vi "2100_Test_Set State_Measure Resistance_Source and Sink.vi"(0 "Semiconductor Module Context":T7, 1 "Script_Info":T3={"Script Name"="WalkingState", "All_Scripts"=[]}, 2 "current range":dbl=1e-05 format="%#_6p", 3 "current level":dbl=1e-05 format="%#_13p", 4 "Instrument_Pins":T6={"SMU_Pins"=["RF1", "RF2", "RF3", "RF4"], "HSDIO_Pins"=["CLK", "SDA"]}, 5 "Error In":errorcluster, 6 "USID":T4, 7 "Master_Register_Data_Array_In":T1 {"Address" format="%.0x"}, 10 "Publishable IDs":string[](array[string])=["RF1", "RF2", "RF3", "RF4"], 11 "Reg_Map_and_Bit_Name":T5={"Reg_Map_Bit_Name"="", "Reg_Map"=[["Reg Addr(0x00)", "7", "6", "5", "4", "3", "2", "1", "0"], ["0", "SPARE", "RF3_SH", "RF2_SH", "RF1_SH", "SPARE", "RF3_RFC", "RF2_RFC", "RF1_RFC"], ["1", "SPARE[7:0]", "", "", "", "", "", "", ""], ["2", "VVAR_EN", "LCM_EN", "RFC_SH", "SPARE", "VARACTOR[3:0]", "", "", ""], ["3", "SW_CTRL1_VIRTUAL[7:0]", "", "", "", "", "", "", ""], ["4", "SW_CTRL1_SWAP", "SW_CTRL1_RBSHIFT[2:0]", "", "", "SW_CTRL1_VSID[3:0]", "", "", ""], ["5", "REG_00_VIRTUAL_MASK[7:0]", "", "", "", "", "", "", ""], ["6", "LOCK_STATUS[1:0]", "", "CLK_DITHER", "FUSES_BURNED", "CLK_IDAC_CAL[3:0]", "", "", ""], ["7", "SPARE[2:0]", "", "", "ODFT_TRIM[4:0]", "", "", "", ""], ["8", "SPARE[2:0]", "", "", "HV_TRIM[4:0]", "", "", "", ""], ["9", "TEST_MUX[2:0]", "", "", "SPARE[1:0]", "", "MEMS_BG_TC[1:0]", "", "MEMSCP_RCM"], ["A", "CP_BOOST_OVRD_EN", "SPARE[2:0]", "", "", "PS_OFF_TIMER[1:0]", "", "PS_ON_TIMER[1:0]", ""], ["0", "", "", "", "", "", "", "", ""], ["D", "Reserved[1:0]", "", "WD_HI_EVENT_CNT[5:0]", "", "", "", "", ""], ["E", "VERSION_ID[7:0]", "", "", "", "", "", "", ""], ["F", "Reserved", "COUNT_200_LSB[6:0]", "", "", "", "", "", ""], ["10", "CLK_DIV2_EN", "Spare", "ODFT_EN", "HV_HYST[4:0]", "", "", "", ""], ["0", "", "", "", "", "", "", "", ""], ["12", "SHORT_FUSE", "FUSE_BURN", "STROBE_EN", "VIO_OK", "RTH[1:0]", "", "FUSE_LOAD_MAN_EN", "FUSE_LOAD"], ["13", "RR_ACK_EN", "Reserved", "ACK_POSITION[1:0]", "", "SuBUS_DRIVE_STRENGTH[3:0]", "", "", ""], ["14", "TM_IO_EN", "TM_IO_SEL", "SuBUS_OVS[1:0]", "", "Reserved[3:0]", "", "", ""], ["15", "Reserved[4:0]", "", "", "", "", "SuBUS_VERSION_PRESENT", "SuBUS_VOLTAGE", "SuBUS_FLAVOR_DEF"], ["16", "PROG_STROBE1_DUR[7:0]", "", "", "", "", "", "", ""], ["17", "PROG_STROBE0_DUR[7:0]", "", "", "", "", "", "", ""], ["18", "Reserved[2:0]", "", "", "EFUSE_SINGLE_ADDR_SEL[4:0]", "", "", "", ""], ["19", "POLL_ADR[4:0]", "", "", "", "", "POLL_BC[2:0]", "", ""], ["1A", "SOFTWARE_RESET", "Reserved[6:0]", "", "", "", "", "", ""], ["1B", "Reserved[7:0]", "", "", "", "", "", "", ""], ["1C", "PWR_MODE_1", "PWR_MODE_0", "TRIGGER_MASK[2:0]", "", "", "TRIGGER[2:0]", "", ""], ["1D", "PRODUCT_ID[7:0]", "", "", "", "", "", "", ""], ["1E", "MANUFACTURER_ID_LSB[7:0]", "", "", "", "", "", "", ""], ["1F", "MANUFACTURER_ID_MSB[3:0]", "", "", "", "USID[3:0]", "", "", ""]]}) -> (15 "Master_Register_Data_Array_Out":T1 {"Address" format="%.0x"}, 19 "Error Out":errorcluster)   [LabVIEW 2013]
uses:
  Controls/USID.ctl
  <vilib>/NI_TestStand_SemiconductorModule/NI_TestStand_Semiconductor_Module.lvlibp/PinMap/General/SemiconductorModuleContext.ctl
  Controls/Master_Reg_Data_Array.ctl
  Controls/Reg_Address_Data.ctl
  <vilib>/NI_TestStand_SemiconductorModule/NI_TestStand_Semiconductor_Module.lvlibp/PinMap/General/Publish/PublishDataDoubleFunctionalTest.vi
  <vilib>/NI_TestStand_SemiconductorModule/NI_TestStand_Semiconductor_Module.lvlibp
panel:
  out "Data_to_LOG":dbl[](array[numeric]) format="%#_6p"
  out "R_Measurements":dbl[][](array[numeric]) format="%#_6p"
  in  "Tab Control":enum32{"Test Info", "Instrument Settings"}(tab)
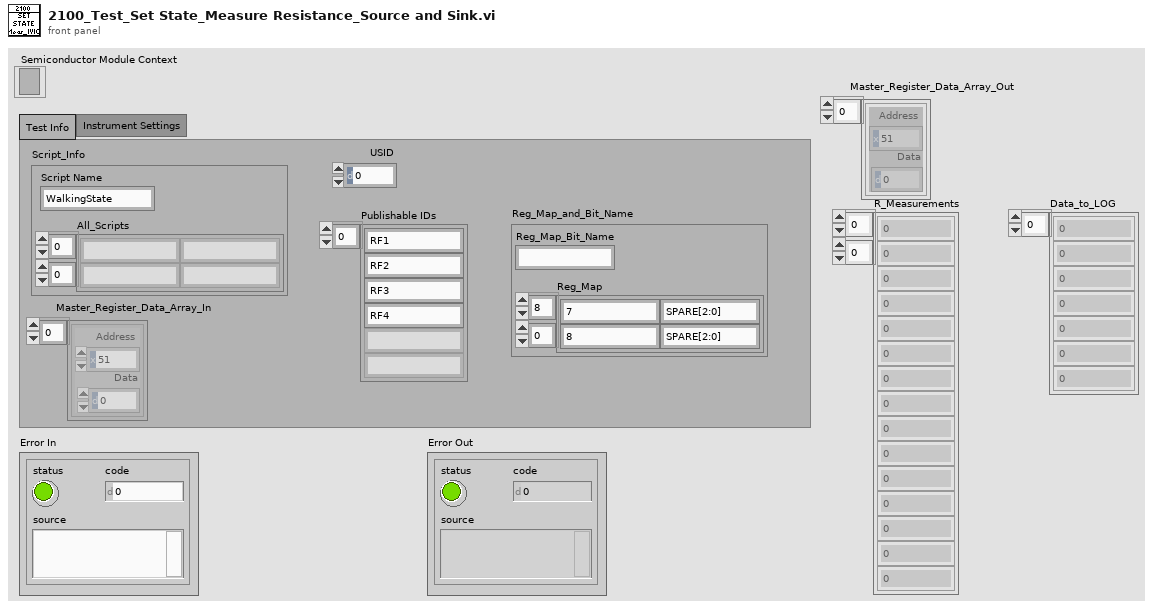
[diagram p1: front panel]
types:
  T1 = typedef "Master_Reg_Data_Array.ctl" = T2[]
  T2 = typedef "Reg_Address_Data.ctl" = cluster{"Address":u8, "Data":u8}
  T3 = cluster{"Script Name":string, "All_Scripts":string[][]}
  T4 = typedef "USID.ctl" = u8
  T5 = cluster{"Reg_Map_Bit_Name":string, "Reg_Map":string[][]}
  T6 = cluster{"SMU_Pins":string[], "HSDIO_Pins":string[]}
  T7 = typedef "NI_TestStand_Semiconductor_Module.lvlibp/SemiconductorModuleContext.ctl" = refnum<k7>
  T8 = typedef "Script Functions_Array.ctl" = enum16{"Reg_Write", "Bit_Write", "Delay", "Read", "Measure"}[]
  T9 = enum16{"Reg_Write", "Bit_Write", "Delay", "Read", "Measure"}
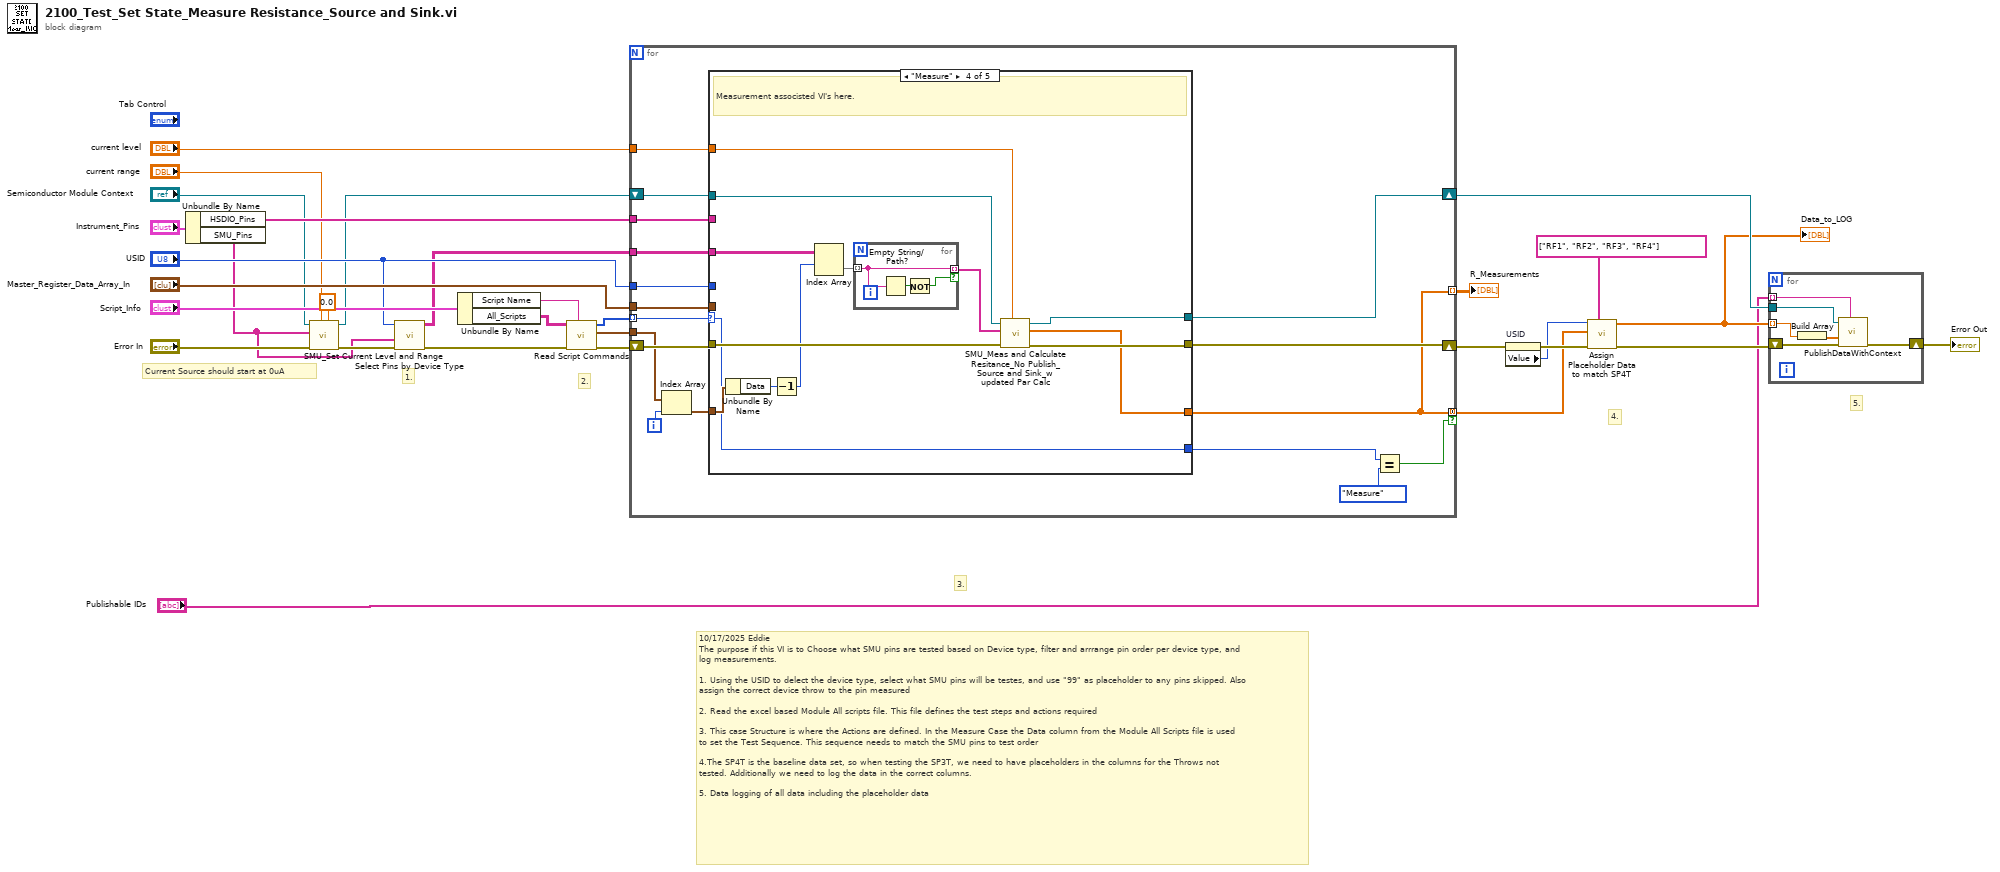
[diagram p0: block diagram]
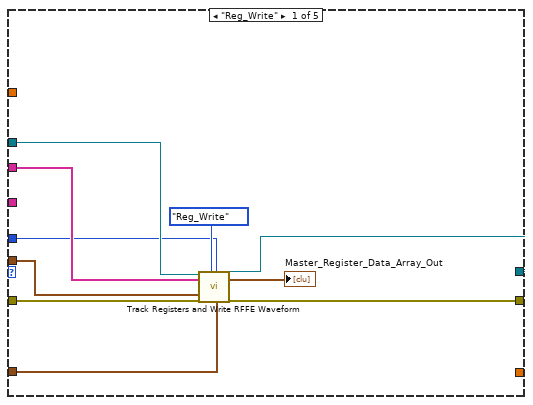
[diagram p2: hidden frame]
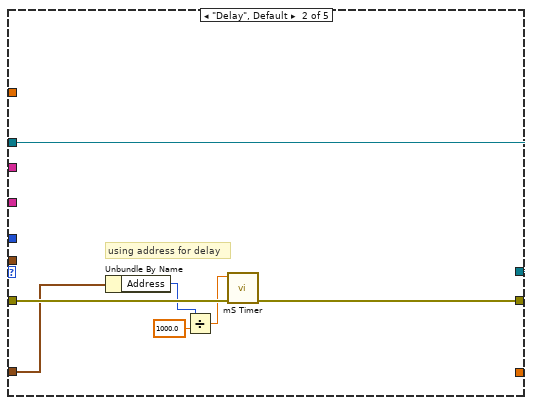
[diagram p3: hidden frame]
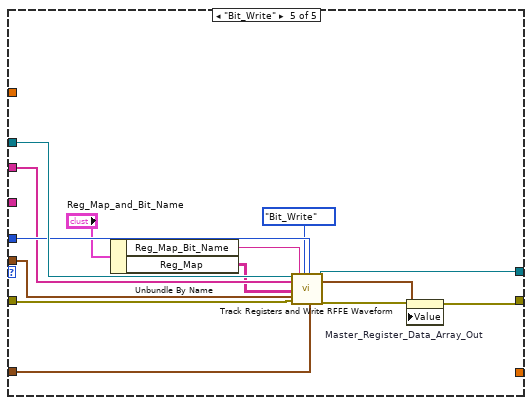
[diagram p5: hidden frame]
diagram:
  # "Current Source should start at 0uA"
  # "4."
  # "10/17/2025 Eddie \nThe purpose if this VI is to Choose what SMU pins are tested based on Device type, filter and arrrange pin order per device type, and log measurements.\n\n1. Using the USID to delect the device type, select what SMU pins will be testes, and use \"99\" as placeholder to any pins skipped. Also assign the correct device throw to the pin measured\n\n2. Read the excel based Module All scripts file. This file defines the test steps and actions required\n\n3. This case Structure is where the Actions are defined. In the Measure Case the Data column from the Module All Scripts file is used to set the Test Sequence. This sequence needs to match the SMU pins to test order\n\n4.The SP4T is the baseline data set, so when testing the SP3T, we need to have placeholders in the columns for the Throws not tested. Additionally we need to log the data in the correct columns.\n\n5. Data logging of all data including the placeholder data"
  # "5."
  # "3."
  # "2."
  # "1."
  n1 = Unbundle By Name("Instrument_Pins") -> ("HSDIO_Pins"=w26:string[], "SMU_Pins"=w1:string[])
  n2 = call "SMU_Set Current Level and Range.vi"("current level"=0.0, "current range"="current range", "error in (no error)"="Error In", "Pins"=w1, "Semiconductor Module Context"="Semiconductor Module Context") -> ("error out"=w8:errorcluster, "Semiconductor Module Context Out"=w6:T7)  [unwired: 5 in]
  n3 = call "Select Pins by Device Type.vi"("error in (no error)"=w8, "Publishable IDs"=w1, "USID"="USID") -> ("error out"=w22:errorcluster, "Pins to Test"=w20:string[][])  [unwired: 7 in]
  n4 = Unbundle By Name("Script_Info") -> ("Script Name"=w23:string, "All_Scripts"=w24:string[][])
  n5 = call "Read Script Commands.vi"("Test Name"=w23, "Error In"=w22, "All_Scripts"=w24) -> ("Error Out"=w29:errorcluster, "Script_Data"=w30:T2[], "Script_Functions"=w31:T8)  [unwired: 5 in, 1 out]
  n6 = for {
    tunnel: "USID" -> [w42]
    tunnel: w31 -> [w41] mode=indexing
    tunnel: w30 -> [w45]
    tunnel: w26 -> [w46]
    shift-right: [w39] -> w15
    shift-left: w29 -> [w48]
    tunnel: "Master_Register_Data_Array_In" -> [w43]
    tunnel: w20 -> [w38]
    shift-right: [w37] -> w18
    shift-left: w6 -> [w47]
    tunnel: [w36] -> w12 mode=concatenating if=w33
    tunnel: [w36] -> w17 mode=indexing
    tunnel: "current level" -> [w32]
    i -> [w40]
    n7 = Index Array(array=w45, index=w40) -> (element=w44:T2)
    n8 = case shown="\"Measure\"" w41 {
      selector: w41 -> [_ _ _ w69 _]
      tunnel: w44 -> [w54 w64 _ w77 w84]
      tunnel: w48 -> [w58 w65 w67 w79 w97]
      tunnel: w42 -> [w51 _ _ _ w91]
      tunnel: w47 -> [w57 w59 w66 w78 w92]
      tunnel: w46 -> [w56 _ _ _ w89]
      tunnel: [w49 w63 w67 w80 w95] -> w39
      tunnel: w43 -> [w53 _ _ _ w88]
      tunnel: w38 -> [_ _ _ w76 _]
      tunnel: [w50 w59 w66 w75 w93] -> w37
      tunnel: [_ _ _ w71 _] -> w36
      tunnel: [_ _ _ w69 _] -> w35
      tunnel: w32 -> [_ _ _ w68 _]
      frame "Reg_Write" {
        n9 = call "Track Registers and Write RFFE Waveform.vi"("Semiconductor Module Context"=w57, "Pins"=w56, "Master_Register_Data_Array_In"=w53, "Error In"=w58, "Script_Functions"=enum16{"Reg_Write", "Bit_Write"}."Reg_Write", "USID"=w51, "Reg_Address_Data"=w54) -> ("Semiconductor Module Context Out"=w50:T7, "Master_Register_Data_Array_Out"=→"Master_Register_Data_Array_Out":T1, "Error Out"=w49:errorcluster)  [unwired: 10 in]
      }
      frame "Delay", Default {
        # "using address for delay"
        n10 = Unbundle By Name(w64) -> ("Address"=w61:u8)
        n11 = Divide(x=w61, y=1000.0) -> (x/y=w60:dbl)
        n12 = call "mS Timer.vi"("Error In"=w65, "Delay(S)"=w60) -> ("Error Out"=w63:errorcluster)  [unwired: 9 in]
      }
      frame "Read" {
        # "Future Dev Code"
      }
      frame "Measure" {
        # "Measurement associsted VI's here."
        n13 = Unbundle By Name(w77) -> ("Data"=w74:u8)
        n14 = Decrement(x=w74) -> (x-1=w70:u8)
        n15 = Index Array(array=w76, index (row)=w70) -> (element=w73:string[])  [unwired: 1 in]
        n16 = for {
          tunnel: w73 -> [w83] mode=indexing
          tunnel: [w83] -> w72 mode=indexing if=w81
          n17 = Empty String/Path?(string/path=w83) -> (empty?=w82:bool)
          n18 = Not(x=w82) -> (.not. x?=w81:bool)
        }
        n19 = call "SMU_Meas and Calculate Resitance_No Publish_Source and Sink_w updated Par Calc.vi"("Current  Level"=w68, "error in (no error)"=w79, "Pins"=w72, "Semiconductor Module Context"=w78) -> ("error Out"=w80:errorcluster, "R Array"=w71:dbl[], "Semiconductor Module Context Out"=w75:T7)  [unwired: 4 in, 1 out]
      }
      frame "Bit_Write" {
        n20 = Unbundle By Name("Reg_Map_and_Bit_Name") -> ("Reg_Map_Bit_Name"=w86:string, "Reg_Map"=w85:string[][])
        n21 = call "Track Registers and Write RFFE Waveform.vi"("Semiconductor Module Context"=w92, "Pins"=w89, "Reg_Map"=w85, "Master_Register_Data_Array_In"=w88, "Error In"=w97, "Reg_Map_Bit_Name"=w86, "Script_Functions"=enum16{"Reg_Write", "Bit_Write"}."Bit_Write", "USID"=w91, "Reg_Address_Data"=w84) -> ("Semiconductor Module Context Out"=w93:T7, "Master_Register_Data_Array_Out"=w94:T1, "Error Out"=w96:errorcluster)  [unwired: 8 in]
        n22 = property on="Master_Register_Data_Array_Out" class="Arr (strict)"(error in=w96, "Value"=w94) -> (error out=w95:errorcluster)  [unwired: 1 in, 1 out]
      }
    }
    n23 = Equal?(x=w35, y=T9."Measure" ("Enum")) -> (x = y?=w33:bool)
  }
  "R_Measurements" <- w17
  n24 = property on="USID" class="DigNum (strict)"(error in=w15) -> (error out=w14:errorcluster, "Value"=w13:T4)  [unwired: 1 in, 1 out]
  n25 = call "Assign Placeholder Data to match SP4T.vi"("SP4T_Pins"=string[] ["RF1", "RF2", "RF3", "RF4"], "error in (no error)"=w14, "Individual_R_Meas"=w12, "USID"=w13) -> ("error out"=w10:errorcluster, "Placeholder_w_Data"=w11:dbl[])  [unwired: 6 in]
  "Data_to_LOG" <- w11
  n26 = for {
    tunnel: "Publishable IDs" -> [w103] mode=indexing
    shift-right: [w102] -> w19
    shift-left: w10 -> [w101]
    tunnel: w18 -> [w99]
    tunnel: w11 -> [w98] mode=indexing
    n27 = Build Array(w98) -> (w100:dbl[])
    n28 = call-poly <vilib>:"PublishDataWithContext.vi"("Published Data Id"=w103, "error in (no error)"=w101, "Data In"=w100, "Semiconductor Module Context"=w99) -> ("error out"=w102:errorcluster)  [unwired: 6 in, 1 out]
  }
  "Error Out" <- w19
